vi "Global1play.vi"() -> ()   [LabVIEW 2014]
panel:
  out "tryg":dbl
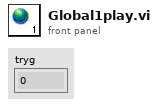
[diagram p1: front panel]
diagram:
